vi "niScope Configure Chan Characteristics.vi"(0 "instrument handle":refnum<k15>, 5 "channels":string="0", 7 "input impedance":u32(ring) items=["1 mega ohm"=0, "50 ohms"=2], 9 "maximum input frequency":dbl caption="max input frequency" format="%.2f", 11 "error in":errorcluster) -> (4 "instrument handle out":refnum<k15>, 15 "error out":errorcluster)   [LabVIEW 2020]
doc: "Configures the properties that control the electrical characteristics of the channel. These properties are the input impedance and the bandwidth."
uses:
  niScope_32.dll
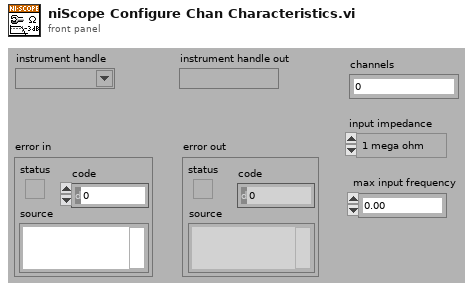
[diagram p1: front panel]
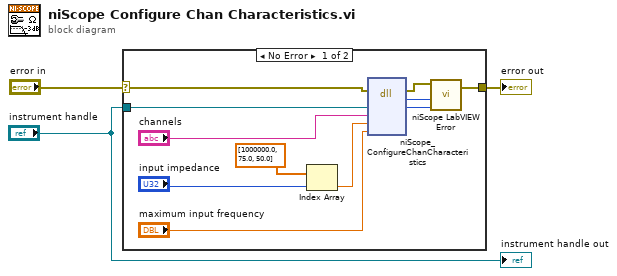
[diagram p0: block diagram]
diagram:
  n1 = case shown="No Error" "error in" {
    selector: "error in" -> [w5 w15]
    tunnel: [w6 w15] -> w2
    tunnel: "instrument handle" -> [w12 _]
    frame No Error {
      n2 = Index Array(array=dbl[] [1000000.0, 75.0, 50.0] ("input impedance arr"), index="input impedance") -> (element=w10:dbl)
      n3 = dll-call lib="niScope_*.*" fn="niScope_ConfigureChanCharacteristics"(error in=w5, "instrument handle"=w12, "channel"="channels", "inputImpedance"=w10, "maxInputFrequency"="maximum input frequency") -> (error out=w4:errorcluster, "status"=w8:i32, "instrument handle"=w7:u32)  [unwired: 5 in, 1 out]
      n4 = call "niScope LabVIEW Error.vi"("instrument handle"=w7, "niScope error code (0)"=w8, "error in (no error)"=w4) -> ("error out"=w6:errorcluster)  [unwired: 2 in]
    }
    frame Error {
    }
  }
  "error out" <- w2
  "instrument handle out" <- "instrument handle"
